vi "SIM Euler.vi"(3 "Simulation data":T1={"continuous integrator"=enum."RK 1 (Euler)", "initial time"=0.1, "final time"=4.0, "step size"=600.0, "proposed step size"=1e-07, "max step size"=0.001, "min step size"=0.0, "discrete time step"=0.0, "max step ratio"=3.0, "Diag Eval Stage"=enum."Major Substep", "Substep Index"=0, "Timestep Index"=10.0, "simulation time"=0.0, "current timestep base"=0.01, "proposed step time"=0.0, "absolute tolerance"=0.0, "relative tolerance"=0.0, "step accepted?"=FALSE, "step complete?"=FALSE, "Halt?"=FALSE, "reset integrator?"=FALSE, "machine epsilon"=6.0, "min float"=0.0, "error"={"status"=FALSE, "code"=0, "source"=""}, "Method Order"=0, "Finished Late [i-1]"=FALSE, "Discrete step?"=FALSE, "NaN and Inf check?"=FALSE, "Final Timestep Index"=0.0, "(maj+disc)or(init)?"=FALSE, "Full Solver Reset"=TRUE, "Execution Mode"=enum."Simulate to Completion", "check vector sizes?"=FALSE, "solver handles zc?"=FALSE, "Simulation Registry"={"Current Idx"=0, "Node Tags"=[], "Node Headers"=[], "Node Data"=[], "Cont State data"={"inputs"=[], "outputs"=[], "reset"=[], "lower limits"=[], "upper limits"=[], "limit types"=[], "reset types"=[], "initial conditions"=[], "reset I.C."=[], "limited?"=[], "State Names"=[]}, "DiscreteInfo"={"tick period (sec)"=0.0, "time (ticks)"=0, "fire?"=[], "registry"={"period (sec)"=[], "skew (sec)"=[], "period (tick)"=[], "skew (tick)"=[]}, "discrete \nblocks?"=FALSE, "steps per tick"=0.0, "steps to tick"=0.0, "discrete \ntick?"=FALSE}, "Disc State data"={"Disc States"=[], "State Names"=[]}, "Registry Error"={"Error Block ID"=0, "code"=0}, "ZC Indices"=[]}, "variable step solver?"=FALSE, "First Substep?"=FALSE, "Continuous States?"=FALSE} {"min float" format="%.1e"; "proposed step size" format="%.1e"; "proposed step time" format="%.1e"; "max step ratio" format="%.1e"; "min step size" format="%.1e"; "machine epsilon" format="%.1e"; "discrete time step" format="%.1e"; "max step size" format="%.1e"; "current timestep base" format="%.1e"; "final time" format="%.1e"; "simulation time" format="%.1e"; "relative tolerance" format="%.1e"; "absolute tolerance" format="%.1e"; "Substep Index" format="%.1e"; "step size" format="%.1e"; "initial time" format="%.1e"}) -> (1 "Simulation data out":T1={"continuous integrator"=enum."RK 1 (Euler)", "initial time"=0.1, "final time"=4.0, "step size"=600.0, "proposed step size"=1e-07, "max step size"=0.001, "min step size"=0.0, "discrete time step"=0.0, "max step ratio"=3.0, "Diag Eval Stage"=enum."Major Substep", "Substep Index"=0, "Timestep Index"=10.0, "simulation time"=0.0, "current timestep base"=0.01, "proposed step time"=0.0, "absolute tolerance"=0.0, "relative tolerance"=0.0, "step accepted?"=FALSE, "step complete?"=FALSE, "Halt?"=FALSE, "reset integrator?"=FALSE, "machine epsilon"=6.0, "min float"=0.0, "error"={"status"=FALSE, "code"=0, "source"=""}, "Method Order"=0, "Finished Late [i-1]"=FALSE, "Discrete step?"=FALSE, "NaN and Inf check?"=FALSE, "Final Timestep Index"=0.0, "(maj+disc)or(init)?"=FALSE, "Full Solver Reset"=TRUE, "Execution Mode"=enum."Simulate to Completion", "check vector sizes?"=FALSE, "solver handles zc?"=FALSE, "Simulation Registry"={"Current Idx"=0, "Node Tags"=[], "Node Headers"=[], "Node Data"=[], "Cont State data"={"inputs"=[], "outputs"=[], "reset"=[], "lower limits"=[], "upper limits"=[], "limit types"=[], "reset types"=[], "initial conditions"=[], "reset I.C."=[], "limited?"=[], "State Names"=[]}, "DiscreteInfo"={"tick period (sec)"=0.0, "time (ticks)"=0, "fire?"=[], "registry"={"period (sec)"=[], "skew (sec)"=[], "period (tick)"=[], "skew (tick)"=[]}, "discrete \nblocks?"=FALSE, "steps per tick"=0.0, "steps to tick"=0.0, "discrete \ntick?"=FALSE}, "Disc State data"={"Disc States"=[], "State Names"=[]}, "Registry Error"={"Error Block ID"=0, "code"=0}, "ZC Indices"=[]}, "variable step solver?"=FALSE, "First Substep?"=FALSE, "Continuous States?"=FALSE} {"min float" format="%.1e"; "proposed step size" format="%.1e"; "proposed step time" format="%.1e"; "max step ratio" format="%.1e"; "min step size" format="%.1e"; "machine epsilon" format="%.1e"; "discrete time step" format="%.1e"; "max step size" format="%.1e"; "current timestep base" format="%.1e"; "final time" format="%.1e"; "simulation time" format="%.1e"; "relative tolerance" format="%.1e"; "absolute tolerance" format="%.1e"; "Substep Index" format="%.1e"; "step size" format="%.1e"; "initial time" format="%.1e"})   [LabVIEW 2017]
uses:
  SIM simulation data.ctl
  SIM integration method.ctl
  SIM diagram eval stage.ctl
  SIMSCR Execution Mode.ctl
  SIM Simulation Registry.ctl
  SIM Registry Node Header.ctl
  SIM Registry Node Record.ctl
  SIM trigger type.ctl
  SIM solver state data.ctl
  SIM limit type.ctl
  SIM discrete data.ctl
  SIM Discrete state data.ctl
  SIM Simulation Registry Error.ctl
  SIM limit signal (array).vi
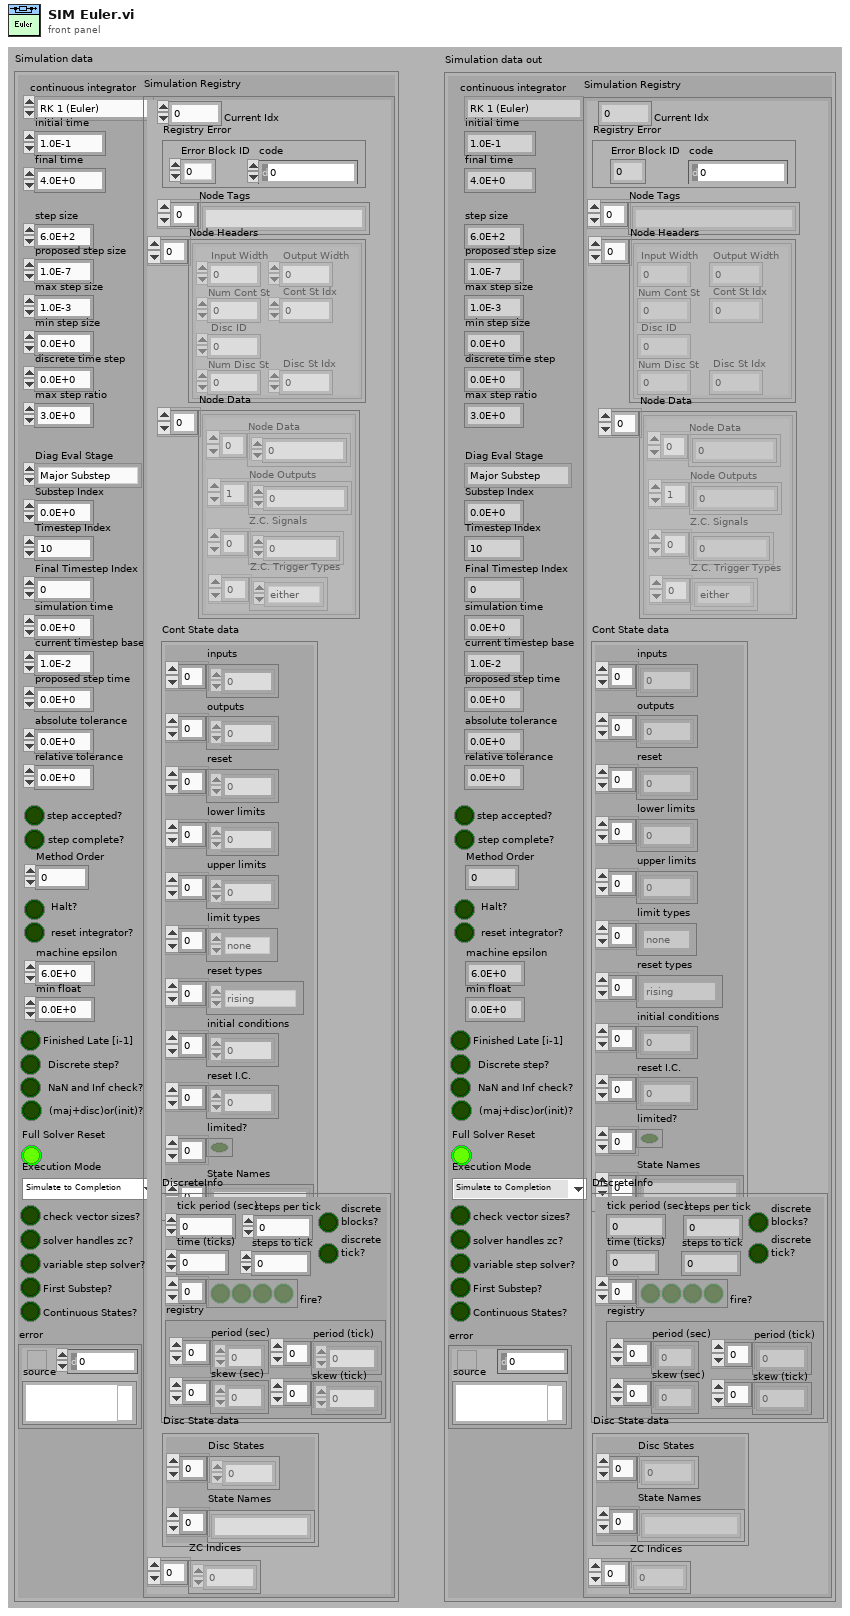
[diagram p1: front panel]
types:
  T1 = typedef "SIM simulation data.ctl" = cluster{"continuous integrator":T2, "initial time":dbl, "final time":dbl, "step size":dbl, "proposed step size":dbl, "max step size":dbl, "min step size":dbl, "discrete time step":dbl, "max step ratio":dbl, "Diag Eval Stage":T3, "Substep Index":i32, "Timestep Index":dbl, "simulation time":dbl, "current timestep base":dbl, "proposed step time":dbl, "absolute tolerance":dbl, "relative tolerance":dbl, "step accepted?":bool, "step complete?":bool, "Halt?":bool, "reset integrator?":bool, "machine epsilon":dbl, "min float":dbl, "error":errorcluster, "Method Order":u32, "Finished Late [i-1]":bool, "Discrete step?":bool, "NaN and Inf check?":bool, "Final Timestep Index":dbl, "(maj+disc)or(init)?":bool, "Full Solver Reset":bool, "Execution Mode":T4, "check vector sizes?":bool, "solver handles zc?":bool, "Simulation Registry":T5, "variable step solver?":bool, "First Substep?":bool, "Continuous States?":bool}
  T2 = typedef "SIM integration method.ctl" = enum16{"RK 1 (Euler)", "Linearizer", "State Query", "Trim Eval", "Adams", "RK 3", "RK 4", "RK 45", "BDF", "RK 2", "RK 23", "Rosenbrock", "Discrete States Only"}
  T3 = typedef "SIM diagram eval stage.ctl" = enum16{"Init", "Minor Substep", "Major Substep", "Final"}
  T4 = typedef "SIMSCR Execution Mode.ctl" = enum16{"Simulate to Completion", "Single Time-Step Simulation (Fixed Step Only)"}
  T5 = typedef "SIM Simulation Registry.ctl" = cluster{"Current Idx":i32, "Node Tags":string[], "Node Headers":T6[], "Node Data":T7[], "Cont State data":T9, "DiscreteInfo":T11, "Disc State data":T12, "Registry Error":T13, "ZC Indices":i32[]}
  T6 = typedef "SIM Registry Node Header.ctl" = cluster{"Input Width":i32, "Disc ID":i32, "Num Cont St":i32, "Cont St Idx":i32, "Num Disc St":i32, "Disc St Idx":i32, "Output Width":i32}
  T7 = typedef "SIM Registry Node Record.ctl" = cluster{"Node Data":dbl[], "Node Outputs":dbl[], "Z.C. Signals":dbl[], "Z.C. Trigger Types":T8[]}
  T8 = typedef "SIM trigger type.ctl" = enum16{"rising", "falling", "either", "none"}
  T9 = typedef "SIM solver state data.ctl" = cluster{"inputs":dbl[], "outputs":dbl[], "reset":dbl[], "lower limits":dbl[], "upper limits":dbl[], "limit types":T10[], "reset types":T8[], "initial conditions":dbl[], "reset I.C.":dbl[], "limited?":bool[], "State Names":string[]}
  T10 = typedef "SIM limit type.ctl" = enum16{"upper", "lower", "both", "none"}
  T11 = typedef "SIM discrete data.ctl" = cluster{"tick period (sec)":dbl, "time (ticks)":i32, "fire?":bool[], "registry":cluster{"period (sec)":dbl[], "skew (sec)":dbl[], "period (tick)":i32[], "skew (tick)":i32[]}, "discrete \nblocks?":bool, "steps per tick":dbl, "steps to tick":dbl, "discrete \ntick?":bool}
  T12 = typedef "SIM Discrete state data.ctl" = cluster{"Disc States":dbl[], "State Names":string[]}
  T13 = typedef "SIM Simulation Registry Error.ctl" = cluster{"Error Block ID":i32, "code":i32}
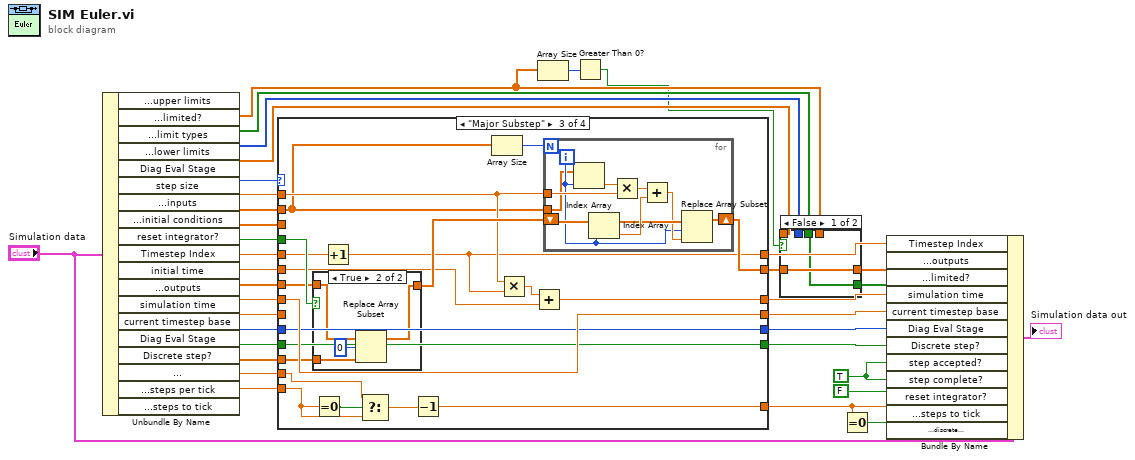
[diagram p0: block diagram]
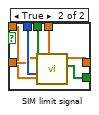
[diagram p2: hidden frame]
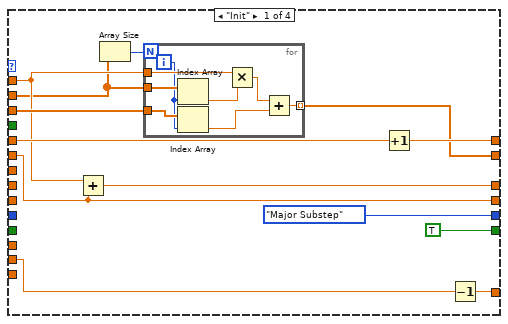
[diagram p3: hidden frame]
diagram:
  w25 = TRUE ("step accepted?")
  n1 = Unbundle By Name("Simulation data") -> ("Simulation Registry.Cont State data.upper limits"=w3:dbl[], "Simulation Registry.Cont State data.limited?"=w16:bool[], "Simulation Registry.Cont State data.limit types"=w15:T10[], "Simulation Registry.Cont State data.lower limits"=w13:dbl[], "Diag Eval Stage"=w34:T3, "step size"=w31:dbl, "Simulation Registry.Cont State data.inputs"=w32:dbl[], "Simulation Registry.Cont State data.initial conditions"=w33:dbl[], "reset integrator?"=w28:bool, "Timestep Index"=w10:dbl, "initial time"=w30:dbl, "Simulation Registry.Cont State data.outputs"=w29:dbl[], "simulation time"=w27:dbl, "current timestep base"=w26:dbl, "Diag Eval Stage"=w9:T3, "Discrete step?"=w22:bool, "Simulation Registry.Cont State data.reset I.C."=w21:dbl[], "Simulation Registry.DiscreteInfo.steps per tick"=w6:dbl, "Simulation Registry.DiscreteInfo.steps to tick"=w7:dbl)
  n2 = case shown="\"Major Substep\"" w34 {
    tunnel: w10 -> [w48 w58 w79 w99]
    tunnel: w33 -> [w43 _ _ _]
    tunnel: w32 -> [w38 _ w70 _]
    tunnel: w31 -> [w42 _ w78 _]
    tunnel: [w40 w59 w80 w103] -> w14
    tunnel: w30 -> [w47 w62 w75 _]
    tunnel: [w47 w62 w77 w102] -> w19
    tunnel: [w46 w62 w74 w102] -> w17
    tunnel: w29 -> [_ w59 w82 w103]
    tunnel: w28 -> [_ _ w83 _]
    tunnel: w27 -> [_ _ w77 _]
    tunnel: w26 -> [_ _ _ w102]
    tunnel: [TRUE ("Discrete step?") w60 w69 w100] -> w20
    tunnel: [SIM_diagram_eval_stage."Major Substep" ("Diag Eval Stage") w61 w72 w101] -> w18
    tunnel: w9 -> [_ w61 w72 w101]
    tunnel: w22 -> [_ w60 w69 w100]
    tunnel: w21 -> [_ _ w73 _]
    tunnel: [w41 w58 w63 w99] -> w8
    tunnel: w6 -> [w36 _ w66 _]
    tunnel: w7 -> [_ w57 w65 w98]
    tunnel: [w37 w57 w64 w98] -> w4
    frame "Init" {
      n3 = Add(x=w42, y=w47) -> (x+y=w46:dbl)
      n4 = Array Size(array=w38) -> (size(s)=w39:i32)
      n5 = for {
        N: w39 -> [_]
        tunnel: w43 -> [w52]
        tunnel: w42 -> [w56]
        tunnel: [w54] -> w40 mode=indexing
        tunnel: w38 -> [w53]
        i -> [w49]
        n6 = Index Array(array=w53, index=w49) -> (element=w51:dbl)
        n7 = Index Array(array=w52, index=w49) -> (element=w50:dbl)
        n8 = Multiply(x=w56, y=w51) -> (x*y=w55:dbl)
        n9 = Add(x=w55, y=w50) -> (x+y=w54:dbl)
      }
      n10 = Increment(x=w48) -> (x+1=w41:dbl)
      n11 = Decrement(x=w36) -> (x-1=w37:dbl)
    }
    frame "Minor Substep" {
    }
    frame "Major Substep" {
      n12 = case shown="True" w83 {
        tunnel: [w93 w97] -> w81
        tunnel: w82 -> [w93 w96]
        tunnel: w73 -> [_ w94]
        frame False {
        }
        frame True {
          n13 = Replace Array Subset(array=w96, new element=w94, index=0) -> (w97:dbl[])
        }
      }
      n14 = Equal To 0?(x=w65) -> (x = 0?=w68:bool)
      n15 = Increment(x=w79) -> (x+1=w63:dbl)
      n16 = Select(t=w66, s=w68, f=w65) -> (s? t:f=w67:dbl)
      n17 = Decrement(x=w67) -> (x-1=w64:dbl)
      n18 = Array Size(array=w70) -> (size(s)=w71:i32)
      n19 = Multiply(x=w78, y=w63) -> (x*y=w76:dbl)
      n20 = Add(x=w76, y=w75) -> (x+y=w74:dbl)
      n21 = for {
        N: w71 -> [_]
        tunnel: w78 -> [w87]
        shift-right: [w88] -> w80
        shift-left: w81 -> [w90]
        tunnel: w70 -> [w84]
        i -> [w85]
        n22 = Index Array(array=w84, index=w85) -> (element=w86:dbl)
        n23 = Index Array(array=w90, index=w85) -> (element=w91:dbl)
        n24 = Multiply(x=w86, y=w87) -> (x*y=w92:dbl)
        n25 = Add(x=w92, y=w91) -> (x+y=w89:dbl)
        n26 = Replace Array Subset(array=w90, new element=w89, index=w85) -> (w88:dbl[])
      }
    }
    frame "Final" {
    }
  }
  n27 = Array Size(array=w3) -> (size(s)=w2:i32)
  n28 = Greater Than 0?(x=w2) -> (x > 0?=w1:bool)
  n29 = case shown="False" w1 {
    tunnel: w16 -> [w104 w112]
    tunnel: w15 -> [_ w111]
    tunnel: w14 -> [w105 w110]
    tunnel: w13 -> [_ w109]
    tunnel: [w105 w108] -> w12
    tunnel: [w104 w107] -> w11
    tunnel: w3 -> [_ w106]
    frame False {
    }
    frame True {
      n30 = call-poly "SIM limit signal.vi"("lower limits"=w109, "upper limits"=w106, "limit types"=w111, "limited? in"=w112, "inputs"=w110) -> ("limited? out"=w107:bool[], "outputs"=w108:dbl[])  [unwired: 5 out]
    }
  }
  n31 = Equal To 0?(x=w4) -> (x = 0?=w5:bool)
  n32 = Bundle By Name(cluster="Simulation data", "Timestep Index"=w8, "Simulation Registry.Cont State data.outputs"=w12, "Simulation Registry.Cont State data.limited?"=w11, "simulation time"=w17, "current timestep base"=w19, "Diag Eval Stage"=w18, "Discrete step?"=w20, "step accepted?"=w25, "step complete?"=w25, "reset integrator?"=FALSE, "Simulation Registry.DiscreteInfo.steps to tick"=w4, "Simulation Registry.DiscreteInfo.discrete \ntick?"=w5) -> (→"Simulation data out":T1)
